vi "MotorPositionGlobals.vi"() -> ()   [LabVIEW 2015]
panel:
  out "Shooting":bool
  out "ClimberSetpoint":dbl
  out "BallHolder":bool=TRUE
  out "RightDriveError":dbl
  out "LeftDriveError":dbl
  out "DisableIntakeControl":bool
  out "IntakeOutput":dbl
  out "TokyoDrift":bool
  out "ManipulatorError":dbl
  out "ManipulatorSetpoint":dbl
  out "WinchError":dbl
  out "TensionerError":dbl
  out "ArmError":dbl
  out "WinchSetpoint":dbl=4900.0
  out "TensionerSetpoint":dbl=-101000.0
  out "ArmSetpoint":dbl=297.0
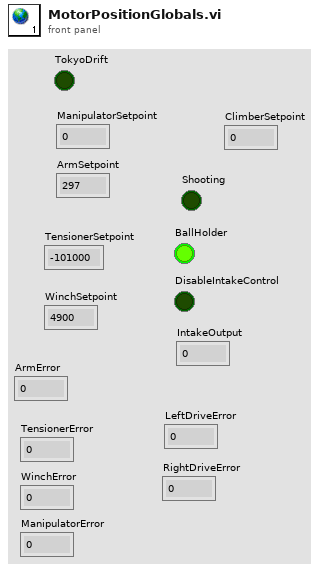
[diagram p1: front panel]
diagram:
